vi "LabVIEWArduino2.vi"() -> ()   [LabVIEW 2020]
uses:
  <vilib>/Instr/_visa.llb/VISA Configure Serial Port (Instr).vi
panel:
  out "match substring":string
  in  "termination char\n(0xA = '\\n' = LF)":u8=10 format="%.0x"
  in  "read byte count":u32
  out "Waveform Graph":dbl[](graph)
  in  "VISA resource name":refnum<visa-resource-name>="COM3"
  in  "data bits (8)":u16=8 min=5 max=8 step=1
  in  "stop bits (10: 1 bit)":u16(ring)=10 items=["1.0"=10, "1.5"=15, "2.0"=20]
  in  "flow control (0:none)":u16(ring) items=["None", "XON/XOFF", "RTS/CTS", "XON/XOFF & RTS/CTS", "DTR/DSR", "XON/XOFF & DTR/DSR"]
  in  "parity (0:none)":enum16{"None", "Odd", "Even", "Mark", "Space"}(ring)
  out "TempArray":dbl[](array[numeric]) caption="Temperature Array"
  out "CurTemp":dbl caption="Current Temperature\n(Celsius)"
  in  "stop":bool
  in  "LabVIEW Stop":bool
  out "LabVIEW Echo":string
  out "Emergency Stop Echo":string
  in  "Emergency Stop!":bool
  out "char sent 2":string
  in  "Decellerate":bool
  in  "Motor Control Duino":refnum<visa-resource-name>
  out "char sent":string
  in  "Accelerate":bool
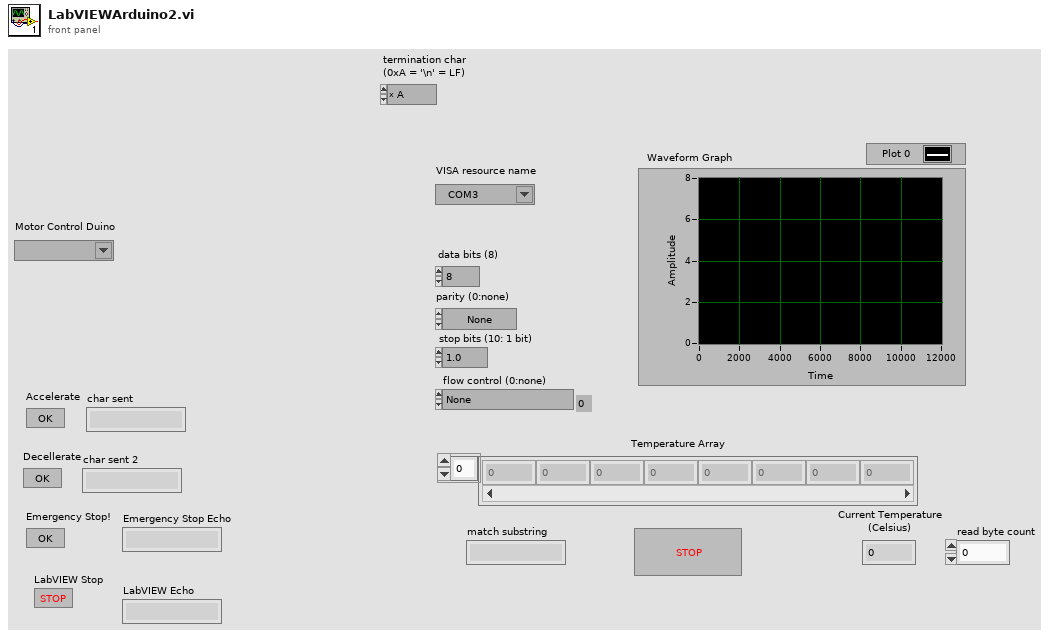
[diagram p1: front panel]
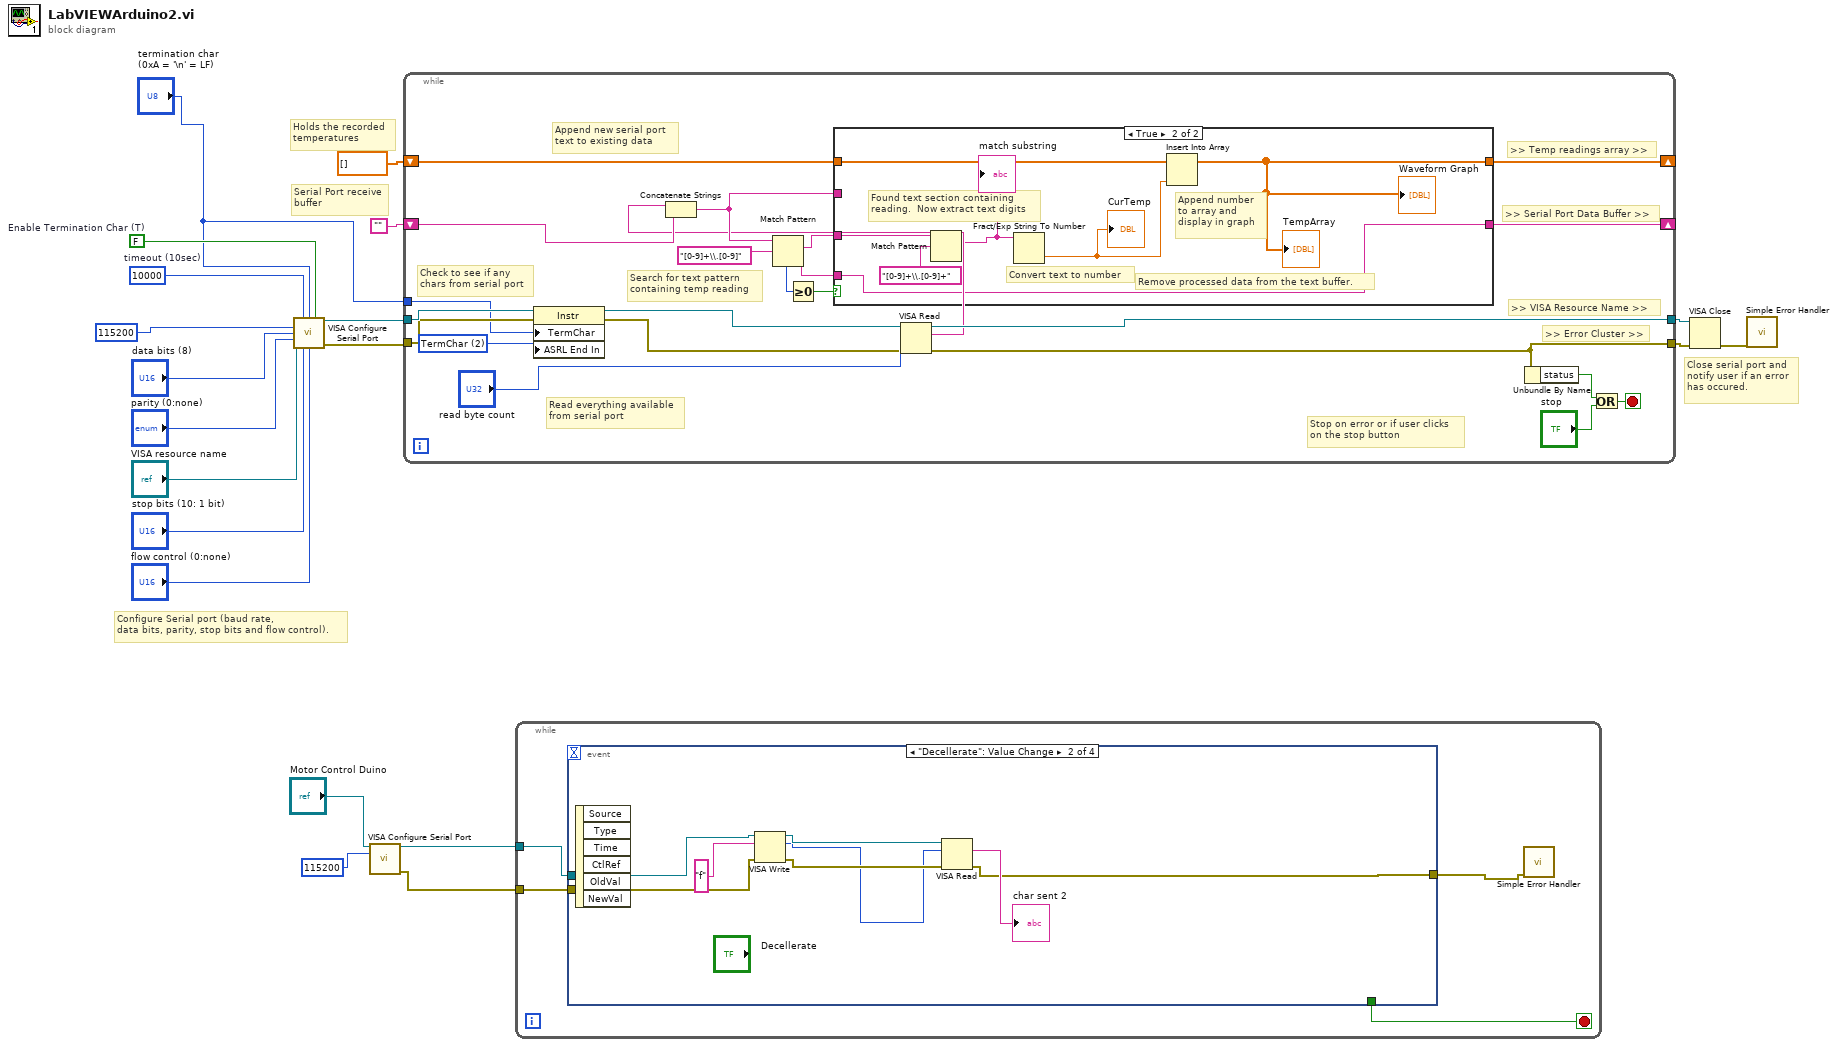
[diagram p0: block diagram]
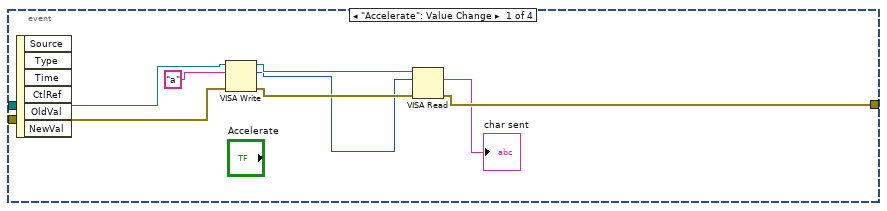
[diagram p3: hidden frame]
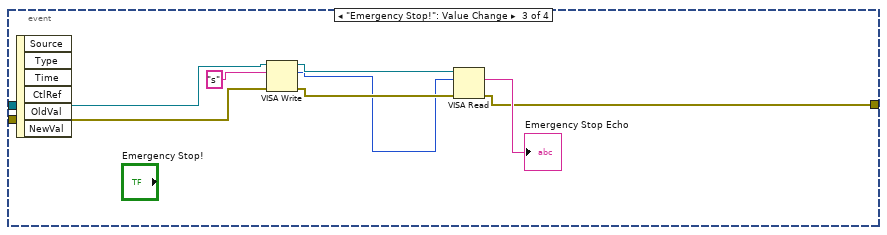
[diagram p4: hidden frame]
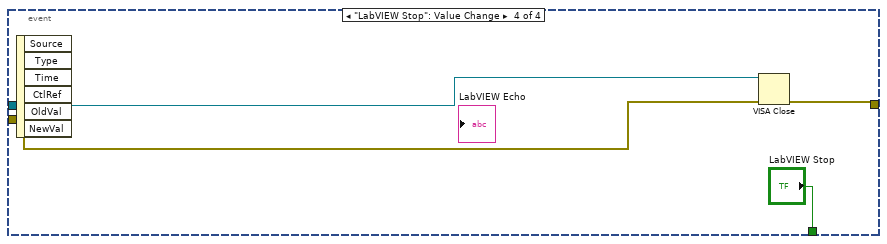
[diagram p5: hidden frame]
diagram:
  w12 = FALSE  # Enable Termination Char (T)
  w13 = u32 10000  # timeout (10sec)
  # "Close serial port and\nnotify user if an error\nhas occured."
  # "Serial Port receive\nbuffer"
  # "Holds the recorded\ntemperatures"
  # "Configure Serial port (baud rate,\ndata bits, parity, stop bits and flow control)."
  n1 = call-poly "VISA Configure Serial Port"("VISA resource name"="VISA resource name", "timeout (10sec)"=w13, "termination char\n(0xA = '\\n' = LF)"="termination char\n(0xA = '\\n' = LF)", "Enable Termination\nChar (T)"=w12, "baud rate (9600)"=u32 115200, "data bits (8)"="data bits (8)", "parity (0:none)"="parity (0:none)", "stop bits (10: 1 bit)"="stop bits (10: 1 bit)", "flow control (0:none)"="flow control (0:none)") -> ("VISA resource name out"=w2:refnum<visa-resource-name>, "error out"=w1:errorcluster)  [unwired: 5 in]
  n2 = call-poly "VISA Configure Serial Port"("VISA resource name"="Motor Control Duino", "baud rate (9600)"=u32 115200) -> ("VISA resource name out"=w20:refnum<visa-resource-name>, "error out"=w19:errorcluster)  [unwired: 12 in]
  n3 = while {
    tunnel: [w41] -> w16
    tunnel: [w43] -> w15
    shift-right: [w35] -> _
    shift-left: "" -> [w42]
    tunnel: w2 -> [w26]
    tunnel: w1 -> [w25]
    shift-right: [w37] -> _
    shift-left: dbl[] [] -> [w36]
    tunnel: "termination char\n(0xA = '\\n' = LF)" -> [w22]
    stop <- w40 stop-if-true
    w21 = u16 2 items=["None", "Last Bit", "TermChar"] ("Serial Settings:End Mode for Reads")
    # "Search for text pattern\ncontaining temp reading"
    # "Append new serial port\ntext to existing data"
    # "Read everything available\nfrom serial port"
    # "Stop on error or if user clicks \non the stop button"
    # ">> Error Cluster >>"
    # ">> VISA Resource Name >>"
    # ">> Temp readings array >>"
    # ">> Serial Port Data Buffer >>"
    # "Check to see if any\nchars from serial port"
    n4 = property class="Instr"(reference=w26, error in=w25, "TermChar"=w22, "ASRL End In"=w21) -> (reference out=w24:refnum<visa-resource-name>, error out=w23:errorcluster)
    n5 = VISA Read(VISA resource name=w24, byte count="read byte count", error in (no error)=w23) -> (VISA resource name out=w43:refnum<visa-resource-name>, read buffer=w28:string, error out=w41:errorcluster)  [unwired: 1 out]
    n6 = Concatenate Strings(w28, w42) -> (w29:string)
    n7 = Match Pattern(string=w29, regular expression="[0-9]+\\.[0-9]") -> (match substring=w31:string, after substring=w30:string, offset past match=w33:i32)  [unwired: 1 in, 1 out]
    n8 = Greater Or Equal To 0?(x=w33) -> (x >= 0?=w32:bool)
    n9 = case shown="True" w32 {
      tunnel: w31 -> [_ w51]
      tunnel: w30 -> [_ w52]
      tunnel: w29 -> [w45 _]
      tunnel: [w45 w52] -> w35
      tunnel: [w44 w46] -> w37
      tunnel: w36 -> [w44 w49]
      frame False {
        # "Did not find text pattern in the buffer.  Try again in the next loop after new data \nhas been received."
      }
      frame True {
        # "Remove processed data from the text buffer."
        # "Append number\nto array and\ndisplay in graph"
        # "Convert text to number"
        # "Found text section containing \nreading.  Now extract text digits"
        n10 = Match Pattern(string=w51, regular expression="[0-9]+\\.[0-9]+") -> (match substring=w50:string)  [unwired: 1 in, 3 out]
        "match substring" <- w50
        n11 = Fract/Exp String To Number(string=w50) -> (number=w47:dbl)  [unwired: 3 in, 1 out]
        "CurTemp" <- w47
        n12 = Insert Into Array(array=w49, new element=w47) -> (w46:dbl[])  [unwired: 1 in]
        "TempArray" <- w46
        "Waveform Graph" <- w46
      }
    }
    n13 = Unbundle By Name(w41) -> ("status"=w39:bool)
    n14 = Or(x=w39, y="stop") -> (x .or. y?=w40:bool)
  }
  n15 = while {
    tunnel: w20 -> [w56]
    tunnel: w19 -> [w55]
    stop <- w53 stop-if-true
    n16 = event shown="[1] \"Decellerate\": Value Change" {
      selector: _ -> [_ _ _ _]
      dyn-events: _ -> [_ _ _ _]
      timeout: _ -> [_ _ _ _]
      tunnel: [w64 w65 w73 w84] -> w54
      tunnel: w56 -> [w60 w67 w75 w83]
      tunnel: w55 -> [w59 w66 w74 w82]
      tunnel: [_ _ _ "LabVIEW Stop"] -> w53
      event "Accelerate": Value Change {
        n17 = event-data() -> ()  [unwired: 1 in, 6 out]
        n18 = VISA Write(VISA resource name=w60, write buffer="a", error in (no error)=w59) -> (VISA resource name out=w62:refnum<visa-resource-name>, return count=w58:u32, error out=w61:errorcluster)
        n19 = VISA Read(VISA resource name=w62, byte count=w58, error in (no error)=w61) -> (read buffer=→"char sent":string, error out=w64:errorcluster)  [unwired: 2 out]
      }
      event "Decellerate": Value Change {
        n20 = event-data() -> ()  [unwired: 1 in, 6 out]
        n21 = VISA Write(VISA resource name=w67, write buffer="f", error in (no error)=w66) -> (VISA resource name out=w71:refnum<visa-resource-name>, return count=w69:u32, error out=w70:errorcluster)
        n22 = VISA Read(VISA resource name=w71, byte count=w69, error in (no error)=w70) -> (read buffer=→"char sent 2":string, error out=w65:errorcluster)  [unwired: 2 out]
      }
      event "Emergency Stop!": Value Change {
        n23 = event-data() -> ()  [unwired: 1 in, 6 out]
        n24 = VISA Write(VISA resource name=w75, write buffer="s", error in (no error)=w74) -> (VISA resource name out=w79:refnum<visa-resource-name>, return count=w77:u32, error out=w78:errorcluster)
        n25 = VISA Read(VISA resource name=w79, byte count=w77, error in (no error)=w78) -> (read buffer=→"Emergency Stop Echo":string, error out=w73:errorcluster)  [unwired: 2 out]
      }
      event "LabVIEW Stop": Value Change {
        n26 = event-data() -> ()  [unwired: 1 in, 6 out]
        n27 = VISA Close(VISA resource name=w83, error in (no error)=w82) -> (error out=w84:errorcluster)
      }
    }
    n28 = call <vilib>:"Simple Error Handler.vi"("error in (no error)"=w54) -> ()  [unwired: 4 in, 5 out]
  }
  n29 = VISA Close(VISA resource name=w15, error in (no error)=w16) -> (error out=w14:errorcluster)
  n30 = call <vilib>:"Simple Error Handler.vi"("error in (no error)"=w14) -> ()  [unwired: 4 in, 5 out]
